vi "Send stack info to conversion.vi"(8 "error in (no error)":errorcluster, 9 "number of frames in":i32, 10 "file path in":path, 11 "DAQOrcaFlash in":refnum<class "DAQOrcaFlash.lvclass">) -> (0 "error out":errorcluster, 3 "DAQOrcaFlash out":refnum<class "DAQOrcaFlash.lvclass">)   [LabVIEW 2012]
uses:
  <vilib>/Distrio/Murmex/Murmex/Murmex.lvclass
  <vilib>/Distrio/Murmex/Murmex/update_cluster.ctl
  DAQOrcaFlash.lvclass
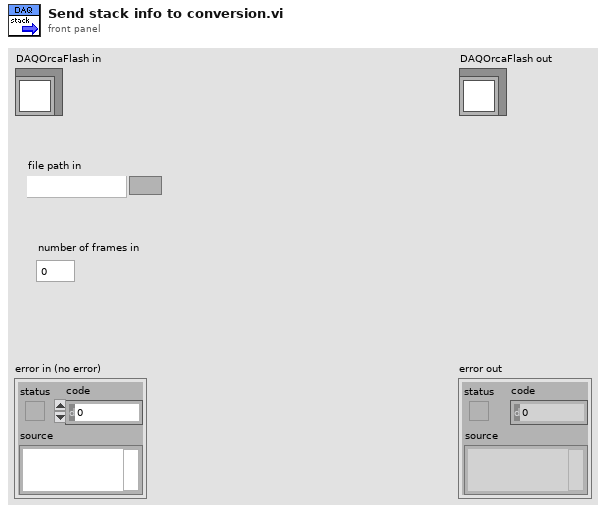
[diagram p1: front panel]
types:
  T1 = typedef "Murmex.lvlib/Murmex.lvclass/update_cluster.ctl" = cluster{"target ID":string, "key chains":string[], "values":variant[]}
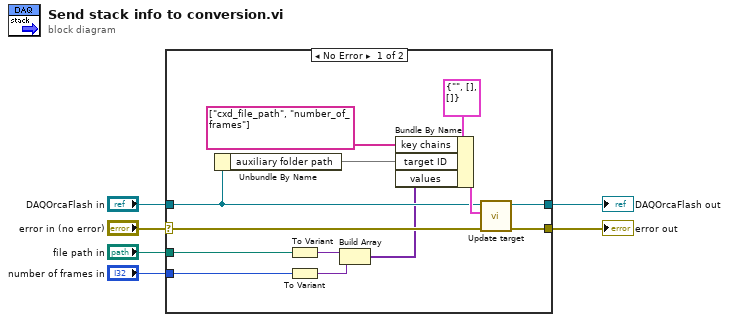
[diagram p0: block diagram]
diagram:
  n1 = case shown="No Error" "error in (no error)" {
    selector: "error in (no error)" -> [w19 w21]
    tunnel: [w18 w21] -> w5
    tunnel: [w17 w20] -> w3
    tunnel: "DAQOrcaFlash in" -> [w14 w20]
    tunnel: "file path in" -> [w11 _]
    tunnel: "number of frames in" -> [w10 _]
    frame No Error {
      n2 = Unbundle By Name(w14) -> ("auxiliary folder path"=w13)
      n3 = To Variant(anything=w11) -> (Variant=w8:variant)
      n4 = To Variant(anything=w10) -> (Variant=w9:variant)
      n5 = Build Array(w8, w9) -> (w7:variant[])
      n6 = Bundle By Name(cluster=T1 {"target ID"="", "key chains"=[], "values"=[]} ("update cluster"), "key chains"=string[] ["cxd_file_path", "number_of_frames"], "target ID"=w13, "values"=w7) -> (w15:T1)
      n7 = call <vilib>:"Update target.vi"("error in (no error)"=w19, "update cluster"=w15, "MurmexBase in"=w14) -> ("error out"=w18:errorcluster, "MurmexBase out"=w17:refnum<class "DAQOrcaFlash.lvclass">)  [unwired: 7 in]
    }
    frame Error {
    }
  }
  "error out" <- w5
  "DAQOrcaFlash out" <- w3
